vi "Insert View.vi"(8 "error in (no error)":errorcluster, 10 "SubPnl Refnum":refnum<vi>, 11 "IViewable in":refnum<class "IViewable.lvclass">) -> (0 "error out":errorcluster, 3 "IViewable out":refnum<class "IViewable.lvclass">)   [LabVIEW 2015, in "IViewable.lvlib" / "IViewable.lvclass"]
uses:
  IViewable.lvclass
  IViewable.lvclass/IViewable.ctl
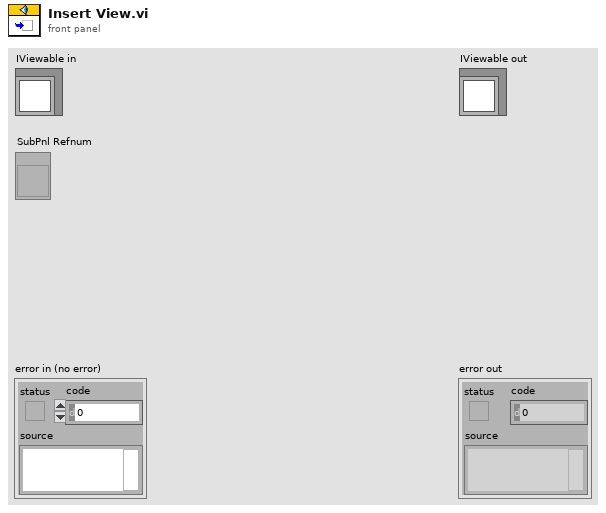
[diagram p1: front panel]
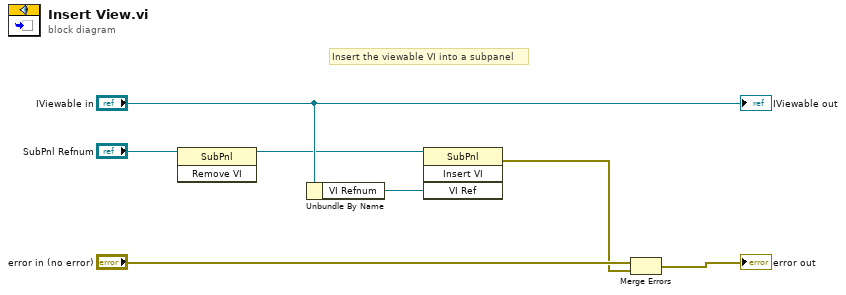
[diagram p0: block diagram]
diagram:
  # "Insert the viewable VI into a subpanel"
  n1 = invoke class="SubPnl" method="Remove VI"(reference="SubPnl Refnum") -> (reference out=w3:refnum<vi>)  [unwired: 2 in, 2 out]
  n2 = Unbundle By Name("IViewable in") -> ("VI Refnum"=w5:refnum<vi>)
  n3 = invoke class="SubPnl" method="Insert VI"(reference=w3, "VI Ref"=w5) -> (error out=w1:errorcluster)  [unwired: 2 in, 3 out]
  n4 = Merge Errors("error in (no error)", w1) -> (→"error out":errorcluster)
  "IViewable out" <- "IViewable in"
